vi "Create.vi"(7 "Root Type (Scalar)":T1, 10 "Value":string) -> (3 "Value Tree out":refnum<class "Value Tree.lvclass">)   [LabVIEW 2020, in "HTTP Server.lvlib" / "Value Tree.lvclass"]
uses:
  Value Tree.lvclass
  Value Tree.lvclass/Value Tree.ctl
  Local Type.ctl
  Local Info.ctl
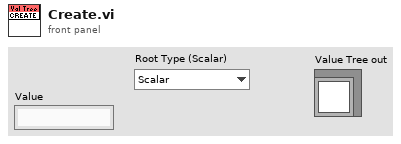
[diagram p1: front panel]
types:
  T1 = typedef "HTTP Server.lvlib/Value Tree.lvclass/Local Type.ctl" = enum16{"Scalar", "Object", "Array"}
  T2 = typedef "HTTP Server.lvlib/Value Tree.lvclass/Local Info.ctl" = cluster{"Type":T1, "Value":string, "Children":string[], "Size":i32}
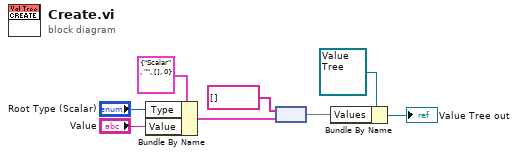
[diagram p0: block diagram]
diagram:
  n1 = Bundle By Name(cluster=T2 {"Type"=enum."Scalar", "Value"="", "Children"=[], "Size"=0} ("Local Info"), "Type"="Root Type (Scalar)", "Value"="Value") -> (w4:T2)
  n2 = node(string[] [], w4) -> (w2:map{string[], T2})
  n3 = Bundle By Name(cluster=refnum<class "Value Tree.lvclass"> refnum ("Value Tree in"), "Values"=w2) -> (→"Value Tree out":refnum<class "Value Tree.lvclass">)
